vi "Event-Stop.vi"(8 "error in (no error)":errorcluster, 10 "Data ref. in":refnum<data-value>, 11 "UI ref. in":refnum<data-value>) -> (0 "error out":errorcluster, 2 "Data ref.":refnum<data-value>, 3 "UI ref.":refnum<data-value>)   [LabVIEW 2013, in "CameraVision.lvlib" / "CV-UI.lvclass"]
uses:
  CV-UI.lvclass
  Main/CV-Main.lvclass
  Main/Main-actions.ctl
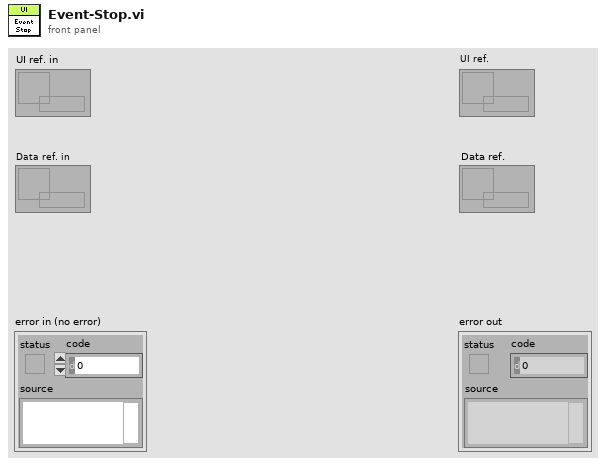
[diagram p1: front panel]
types:
  T1 = typedef "CameraVision.lvlib/CV-Main.lvclass/Main-actions.ctl" = enum16{"Idle", "Initialize", "Load defaults", "Update settings", "Check settings", "Save settings", "Save settings with dialog", "Load settings", "Load data", "Activate", "Start", "Wait for start signal", "Acquire & process", "Iterate", "Stop", "Refresh display", "Refresh status", "View camera settings", "View grabber settings", "Exit"}
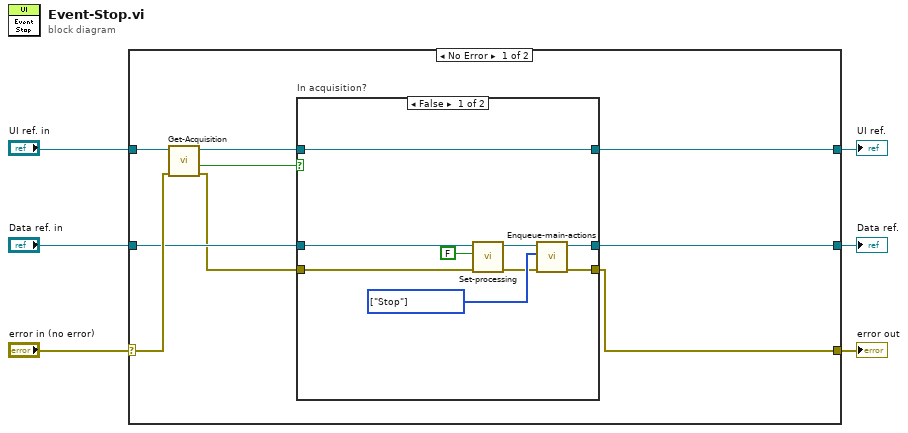
[diagram p0: block diagram]
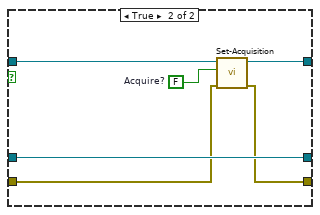
[diagram p2: hidden frame]
diagram:
  n1 = case shown="No Error" "error in (no error)" {
    selector: "error in (no error)" -> [w10 w33]
    tunnel: [w12 w33] -> w5
    tunnel: [w15 w32] -> w3
    tunnel: "UI ref. in" -> [w13 w32]
    tunnel: "Data ref. in" -> [w9 w31]
    tunnel: [w14 w31] -> w1
    frame No Error {
      n2 = call "Get-Acquisition.vi"("error in (no error)"=w10, "UI ref. in"=w13) -> ("error out"=w8:errorcluster, "Acquisition"=w7:bool, "UI ref."=w11:refnum<data-value>)  [unwired: 7 in]
      n3 = case "In acquisition?" shown="False" w7 {
        tunnel: w11 -> [w24 w29]
        tunnel: w9 -> [w17 w30]
        tunnel: [w24 w28] -> w15
        tunnel: [w21 w30] -> w14
        tunnel: w8 -> [w18 w26]
        tunnel: [w23 w25] -> w12
        frame False {
          w22 = T1[] [enum."Stop"] items=["Idle", "Initialize", "Load defaults", "Update settings", "Check settings", "Save settings", "Save settings with dialog", "Load settings", "Load data", "Activate", "Start", "Wait for start signal", "Acquire & process", "Iterate", "Stop", "Refresh display", "Refresh status", "View camera settings", "View grabber settings", "Exit"] ("State array")
          n4 = call "Set-processing.vi"("error in (no error)"=w18, "Processing"=FALSE ("Stop"), "Data ref. in"=w17) -> ("error out"=w19:errorcluster, "Data ref."=w20:refnum<data-value>)  [unwired: 7 in]
          n5 = call "Enqueue-main-actions.vi"("error in (no error)"=w19, "State array"=w22, "Data ref. in"=w20) -> ("error out"=w23:errorcluster, "Data ref."=w21:refnum<data-value>)  [unwired: 6 in, 1 out]
        }
        frame True {
          w27 = FALSE  # Acquire?
          n6 = call "Set-Acquisition.vi"("error in (no error)"=w26, "Acquisition"=w27, "UI ref. in"=w29) -> ("error out"=w25:errorcluster, "UI ref."=w28:refnum<data-value>)  [unwired: 7 in]
        }
      }
    }
    frame Error {
    }
  }
  "error out" <- w5
  "Data ref." <- w1
  "UI ref." <- w3
